vi "Stop.vi"(8 "error in":errorcluster, 11 "Virtual Instrument in":refnum<class "Virtual Instrument.lvclass">) -> (0 "error out":errorcluster, 3 "Virtual Instrument out":refnum<class "Virtual Instrument.lvclass">)   [LabVIEW 2024, in "HAL.lvlib" / "Virtual Instrument.lvclass"]
uses:
  Virtual Instrument.lvclass
  Virtual Instrument.lvclass/Virtual Instrument.ctl
  Instrument/Instrument.lvclass
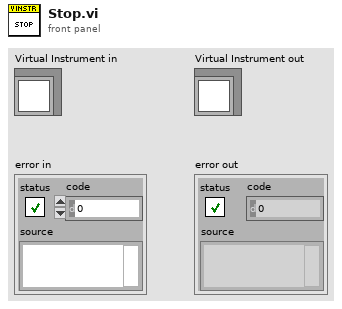
[diagram p1: front panel]
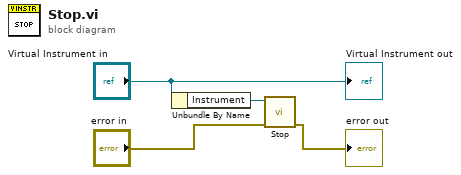
[diagram p0: block diagram]
diagram:
  n1 = Unbundle By Name("Virtual Instrument in") -> ("Instrument"=w3:refnum<class "Instrument.lvclass">)
  n2 = call "Stop.vi"("Error In"="error in", "reference in"=w3) -> ("Error Out"=→"error out":errorcluster)  [unwired: 8 in, 1 out]
  "Virtual Instrument out" <- "Virtual Instrument in"
